vi "Init Model.vi"(8 "error in":errorcluster, 11 "Notifiers in":T1) -> (0 "error out":errorcluster, 3 "Notifiers out":T1)   [LabVIEW 2014, in "Model.lvlib"]
uses:
  Model.lvlib
  support/Message Queue/Message Queue.lvlib
  Support/Message Queue/Enqueue Message (Single).vi
  PLC/PLC.lvlib
  Support/Notifiers/Notifiers.ctl
  Support/Notifiers/Notifiers.lvlib
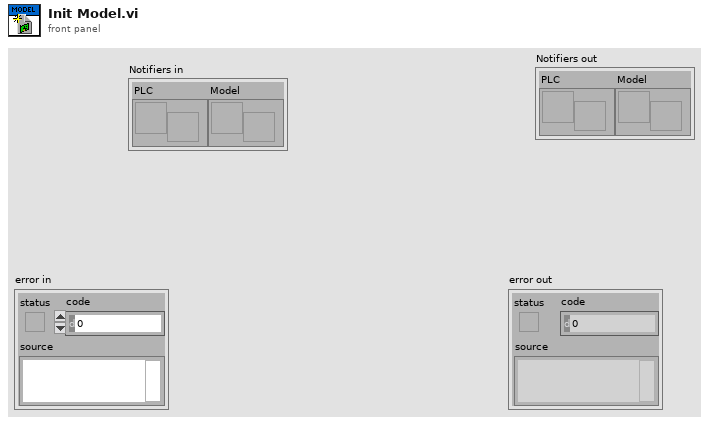
[diagram p1: front panel]
types:
  T1 = typedef "Notifiers.lvlib/Notifiers.ctl" = cluster{"PLC":refnum<notifier>, "Model":refnum<notifier>}
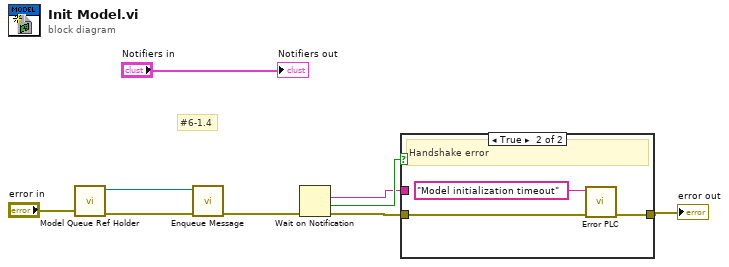
[diagram p0: block diagram]
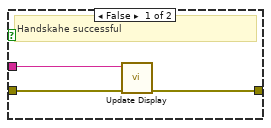
[diagram p2: hidden frame]
diagram:
  # "#6-1.4"
  n1 = call "Model Queue Ref Holder.vi"("error in"="error in") -> ("error out"=w5:errorcluster, "Input Message Queue"=w4:refnum<queue>)  [unwired: 9 in]
  n2 = call-poly "Enqueue Message.vi"("error in (no error)"=w5, "Message Queue"=w4) -> ("error out"=w7:errorcluster)  [unwired: 8 in, 1 out]
  n3 = Wait on Notification(error in (no error)=w7) -> (notification=w6:string, timed out?=w8:bool, error out=w9:errorcluster)  [unwired: 3 in, 1 out]
  n4 = case shown="True" w8 {
    tunnel: w9 -> [w11 w14]
    tunnel: [w10 w13] -> w3
    tunnel: w6 -> [w12 _]
    frame False {
      # "Handskahe successful"
      n5 = call "Update Display.vi"("error in"=w11, "Message string"=w12) -> ("error out"=w10:errorcluster)  [unwired: 9 in]
    }
    frame True {
      # "Handshake error"
      n6 = call "Error PLC.vi"("error in"=w14, "String"="Model initialization timeout" ("Message")) -> ("error out"=w13:errorcluster)  [unwired: 9 in]
    }
  }
  "error out" <- w3
  "Notifiers out" <- "Notifiers in"
